vi "Transport_Read_Plot_2.vi"(6 "default (0 dbl)":ext format="%.2e", 9 "Transport Graph Properties":T1={"Transport Line Size"=0, "Transport Line Color"=16774656} {"Transport Line Size" items=["Extra Small", "Small", "Medium", "Large", "Extra Large"]}, 10 "Transport File Path":path) -> (1 "Array 2":ext[][](array[numeric]), 2 "Array":ext[][](array[numeric]), 3 "Transport File":path, 4 "Transport":cluster{ext[], ext[]}[](graph))   [LabVIEW 2015]
uses:
  <vilib>/Utility/file.llb/Read Delimited Spreadsheet (string).vi
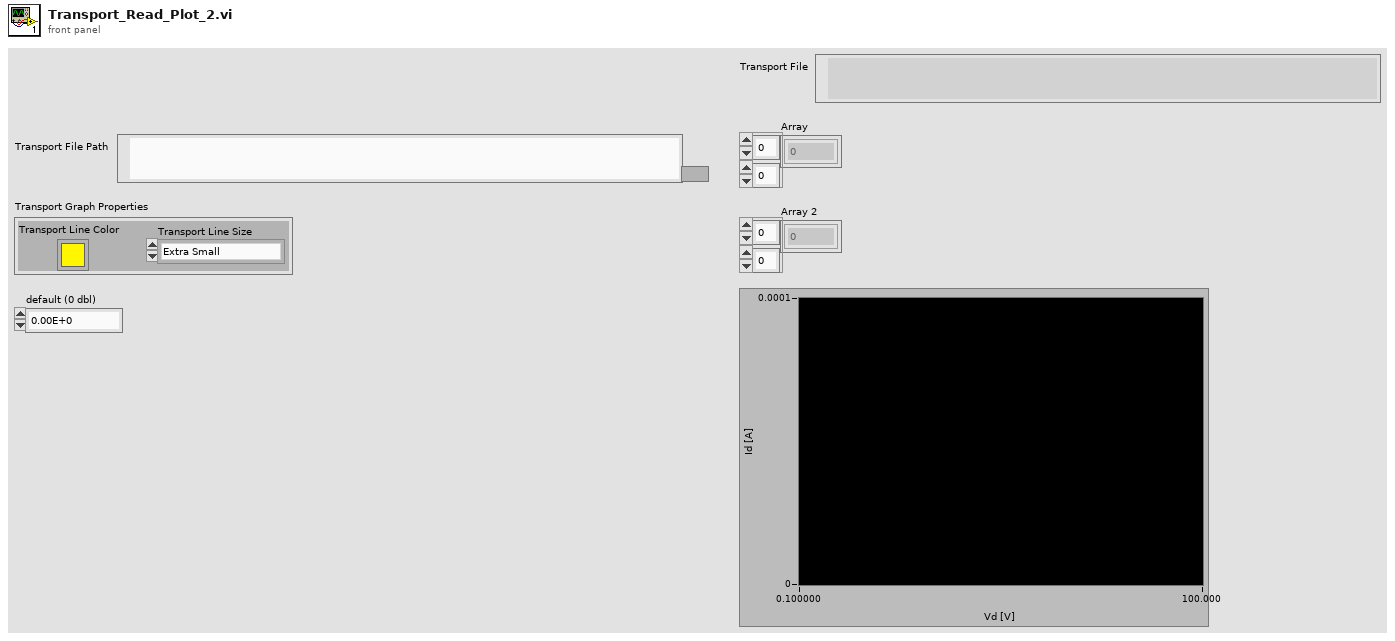
[diagram p1: front panel]
types:
  T1 = cluster{"Transport Line Size":u16, "Transport Line Color":u32}
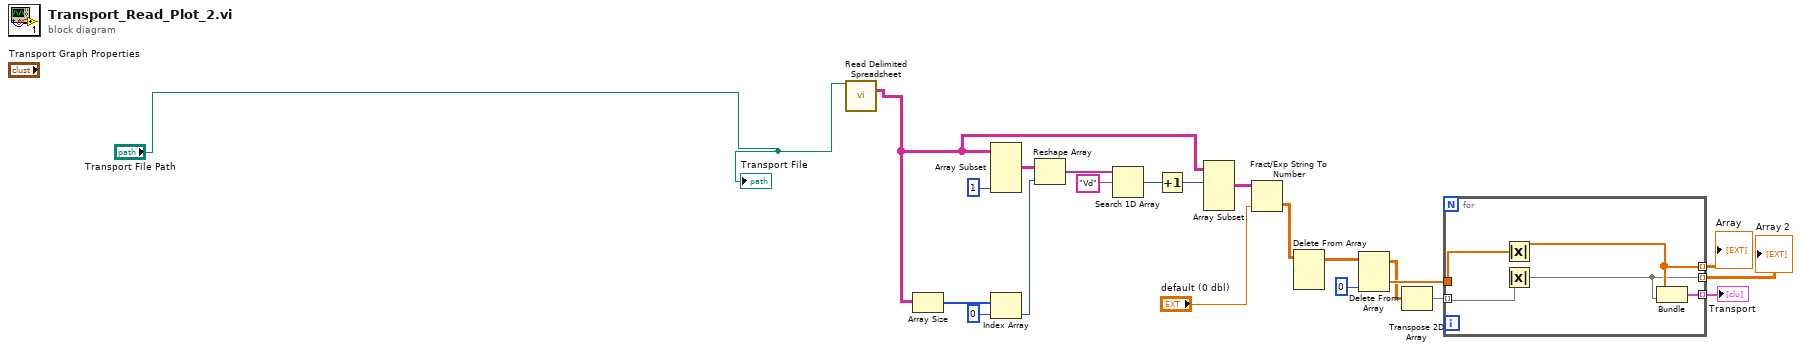
[diagram p0: block diagram]
diagram:
  n1 = call-poly <vilib>:"Read Delimited Spreadsheet.vi"("file path (dialog if empty)"="Transport File Path") -> ("all rows"=w19:string[][])  [unwired: 9 in, 5 out]
  n2 = Array Size(array=w19) -> (size(s)=w1:i32[])
  n3 = Array Subset(array=w19, length (col)=1) -> (w5:string[][])  [unwired: 3 in]
  n4 = Index Array(array=w1, index=0) -> (element=w11:i32)
  n5 = Reshape Array(w5, w11) -> (w6:string[])
  n6 = Search 1D Array(1D array=w6, element="Vd") -> (index of element=w7:i32)  [unwired: 1 in]
  n7 = Increment(x=w7) -> (x+1=w8:i32)
  n8 = Array Subset(array=w19, index (row)=w8) -> (w10:string[][])  [unwired: 3 in]
  n9 = Fract/Exp String To Number(string=w10, default (0 dbl)="default (0 dbl)") -> (number=w16:ext[][])  [unwired: 2 in, 1 out]
  n10 = Delete From Array(array=w16) -> (array with subset deleted=w17:ext[][])  [unwired: 3 in, 1 out]
  n11 = Delete From Array(array=w17, index (col)=0 ("Deaktivierter Index (Spalte)")) -> (deleted portion=w14:ext[], array with subset deleted=w13:ext[][])  [unwired: 2 in]
  n12 = Transpose 2D Array(2D array=w13) -> (transposed array=w12:ext[][])
  n13 = for {
    tunnel: w14 -> [w26]
    tunnel: w12 -> [w25] mode=indexing
    tunnel: [w27] -> w18 mode=indexing
    tunnel: [w24] -> w21 mode=indexing
    tunnel: [w23] -> w22 mode=indexing
    n14 = Absolute Value(x=w26) -> (abs(x)=w24:ext[])
    n15 = Absolute Value(x=w25) -> (abs(x)=w23:ext[])
    n16 = Bundle(w24, w23) -> (w27:cluster{ext[], ext[]})  [unwired: 1 in]
  }
  "Transport" <- w18
  "Array" <- w21
  "Array 2" <- w22
  "Transport File" <- "Transport File Path"
